vi "Multiprocessing_VI.vi"() -> ()   [LabVIEW 2022 SP3]
uses:
  <vilib>/Analysis/baseanly.llb/Mean (DBL).vi
  <vilib>/DAQmx/read.llb/DAQmx Read (Analog 1D Wfm NChan NSamp).vi
  STOP_GLOBAL.vi
  <vilib>/DAQmx/configure/timing.llb/DAQmx Timing (Sample Clock).vi
  <vilib>/addons/control/pid/pid.llb/PID Gain Schedule (DBL).vi
  <vilib>/DAQmx/miscellaneous.llb/DAQmx Fill In Error Info.vi
  <resource>/objmgr/daqmx.rc
  <vilib>/addons/control/pid/NI_PID_pid.lvlib
  <vilib>/Analysis/NI_AALBase.lvlib
panel:
  out "Angle":dbl
  in  "Voltage 2":dbl
  out "Angle Sensor":dbl[](graph)
  in  "Manual Angle Control":dbl
  out "Voltage":dbl
  out "Voltage Command Output":dbl[](graph)
  out "VoltageSent":dbl
  out "Ball Valve Angle Command":dynamicdata(graph)
  in  "Ignition":bool
  in  "Stepper Voltage":ext format="%_3g"
  out "Chamber Pressure LocalVar":dynamicdata(graph)
  out "PID gains out":T1={"proportional gain (Kc)"=1.0, "integral time (Ti, min)"=0.01, "derivative time (Td, min)"=0.0} {"derivative time (Td, min)" format="%.3f"; "integral time (Ti, min)" format="%.5f"; "proportional gain (Kc)" format="%.3f"}
  out "Process Variable vs Setpoint":dynamicdata(graph)
  out "Output":dbl(slide)=30.8641975308642 scale=0.0..5.067 scale format="%.1f"
  in  "Automatic":bool=TRUE
  out "Servo/Step Voltage":dbl[](array[numeric])
  in  "SP":dbl
  in  "MV":dbl(slide)=30.8641975308642 scale=0.0..5.067 scale format="%.1f"
  in  "Stop All":bool
  out "D.C. Delay":dbl
  out "AI7":dynamicdata(graph)
  out "Time":dbl
  out "Inlet Thermocouple":cluster{dbl[], dbl[]}(graph)
  out "Inlet Thermocouple":dynamicdata(graph)
  out "Flow Meter Thermocouple":dynamicdata(graph)
  out "Flow Meter Thermocouple":cluster{dbl[], dbl[]}(graph)
  out "Supply P. Thermocouple":cluster{dbl[], dbl[]}(graph)
  out "Supply P. Thermocouple":dynamicdata(graph)
  out "Thrust 3":cluster{dbl[], dbl[]}(graph)
  out "Thrust 2":cluster{dbl[], dbl[]}(graph)
  out "Rocket Thrust":cluster{dbl[], dbl[]}(graph)
  out "LC2":dynamicdata(graph)
  out "Rocket Thrust LC1":dynamicdata(graph)
  out "LC3":dynamicdata(graph)
  out "Waiting \nfor Start":bool=TRUE
  in  "Start VI":bool
  out "SampClk.Rate":dbl
  in  "Sample Number":i32=100
  in  "Channel Control":bool[](array[boolean])
  in  "Rate":dbl=1000.0 format="%0.2f"
  out "AI7":cluster{dbl[], dbl[]}(graph)
  out "Vol Flow L/min":dynamicdata(graph)
  out "Process Variable vs Setpoint":cluster{dbl[], dbl[]}[](graph)
  in  "Filename":path=path "C:/1. Rocket Research Project/CollectedData/Plots/TestingData.lvm"
  in  "PID gain schedule":T2(array[cluster])=[{"PID gains"={"proportional gain (Kc)"=1.0, "integral time (Ti, min)"=0.01, "derivative time (Td, min)"=0.0}, "max value"=100.0}] {"max value" format="%.2f"; "PID gains"."derivative time (Td, min)" format="%.3f"; "PID gains"."integral time (Ti, min)" format="%.3f"; "PID gains"."proportional gain (Kc)" format="%.3f"}
  in  "Collect?":bool=TRUE caption="Enable"
  out "Vol Flow":cluster{dbl[], dbl[]}(graph)
  out "Chamber Pressure":cluster{dbl[], dbl[]}(graph)
  out "Inlet Pressure":cluster{dbl[], dbl[]}(graph)
  out "Flow Meter Pressure":cluster{dbl[], dbl[]}(graph)
  out "Supply Pressure":cluster{dbl[], dbl[]}(graph)
  out "Supply Pressure":dynamicdata(graph)
  out "Inlet Pressure":dynamicdata(graph)
  out "Line Pressure":dynamicdata(graph)
  out "Chamber Pressure PSI":dynamicdata(graph)
  out "Output Clock Rate":dbl
  out "For loop iterations":i32
  out "error out":errorcluster
  out "Iterations":i32
  out "Angle Sensor":dynamicdata(graph)
  out "P.T. 5":dynamicdata(graph)
  # "Temperature Channels"
  # "Thrust Channels"
  # "DAQ Configuration"
  # "AI 0 - Supply Pressure"
  # "AI 1 - Flow Meter Pressure"
  # "AI 2 - Inlet Pressure"
  # "AI 3 - Chamber Pressure"
  # "AI 4 - Differential Pressure"
  # "AI 5 - Volumetric Flow"
  # "AI 6 - Angle Sensor"
  # "AI 7"
  # "Load Cell 1 Right"
  # "Load Cell 2 Left"
  # "Thrust Channel 3"
  # "TC1 - Supply P. Thermocouple"
  # "TC2 - Flow Meter Thermocouple"
  # "TC3 - Inlet Thermocouple"
  # "Pressure Channels"
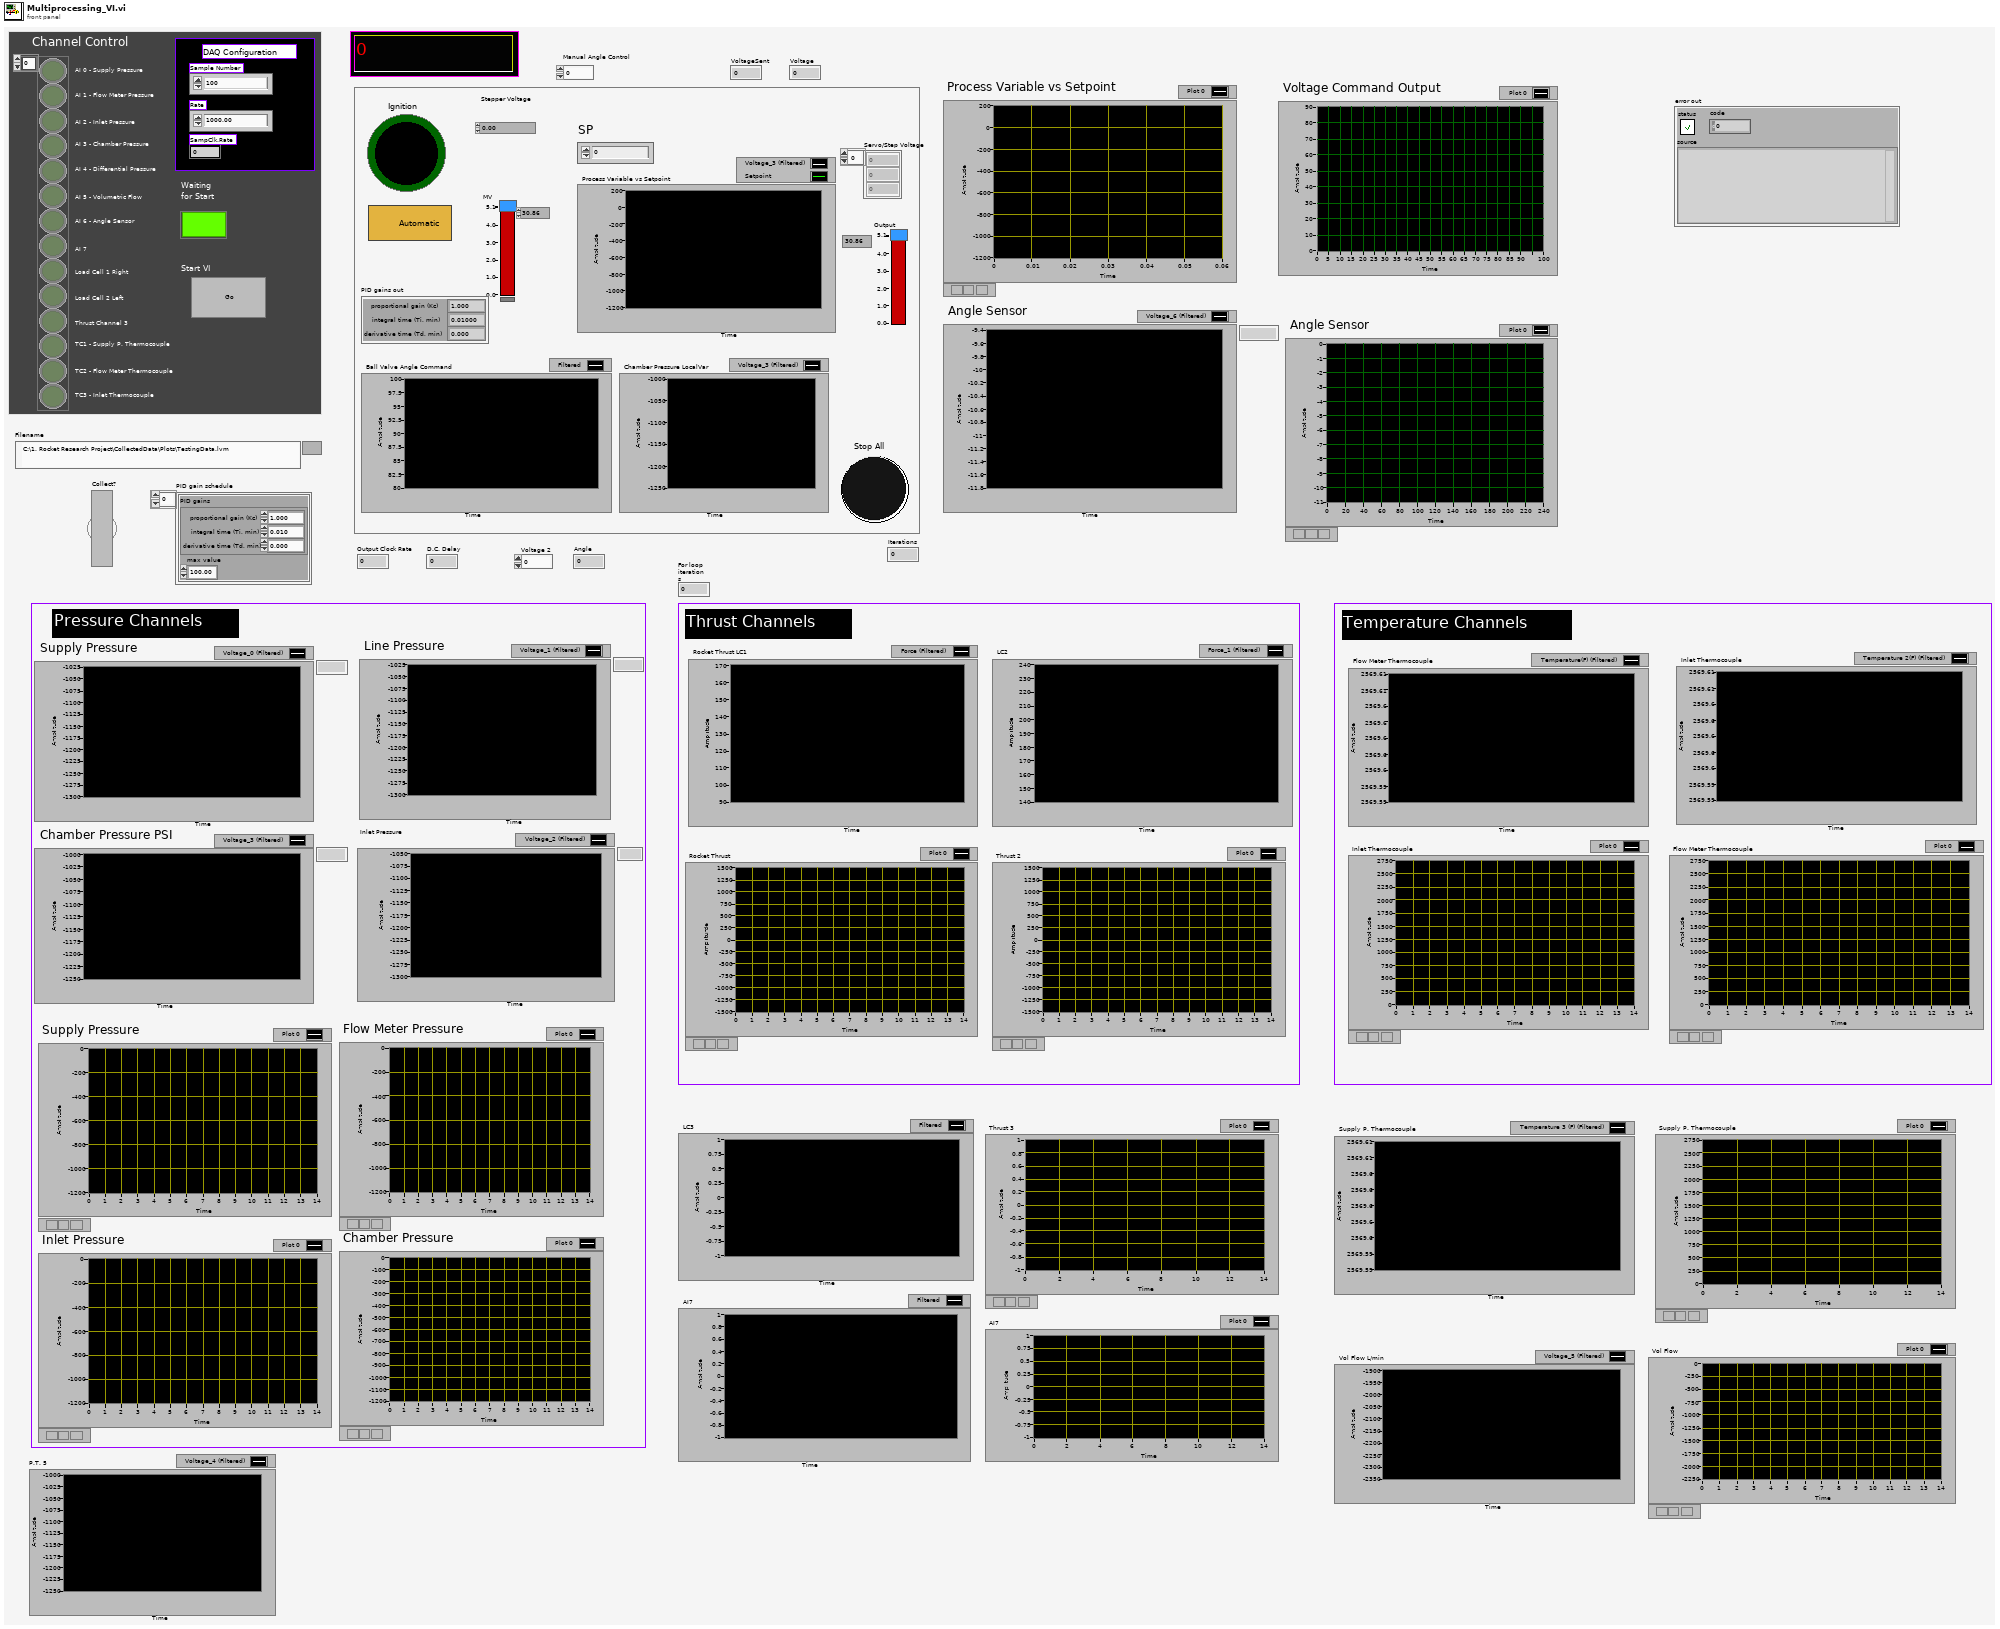
[diagram p1: front panel]
types:
  T1 = cluster{"proportional gain (Kc)":dbl, "integral time (Ti, min)":dbl, "derivative time (Td, min)":dbl}
  T2 = cluster{"PID gains":cluster{"proportional gain (Kc)":dbl, "integral time (Ti, min)":dbl, "derivative time (Td, min)":dbl}, "max value":dbl}[]
  T3 = cluster{"PID gains":cluster{"Kc":dbl, "Ti":dbl, "Td":dbl}, "max value":dbl}[]
  T4 = cluster{"Modulus":dbl, "Number of\nComplete Cycles":dbl}
  T5 = cluster{"Dynamic Data":dynamicdata, "Dynamic Data":dynamicdata, "Dynamic Data":dynamicdata, "Dynamic Data":dynamicdata, "Dynamic Data":dynamicdata, "Dynamic Data":dynamicdata, "Dynamic Data":dynamicdata, "Dynamic Data":dynamicdata, "Dynamic Data":dynamicdata, "Dynamic Data":dynamicdata, "Dynamic Data":dynamicdata, "Dynamic Data":dynamicdata, "Dynamic Data":dynamicdata, "Dynamic Data":dynamicdata}
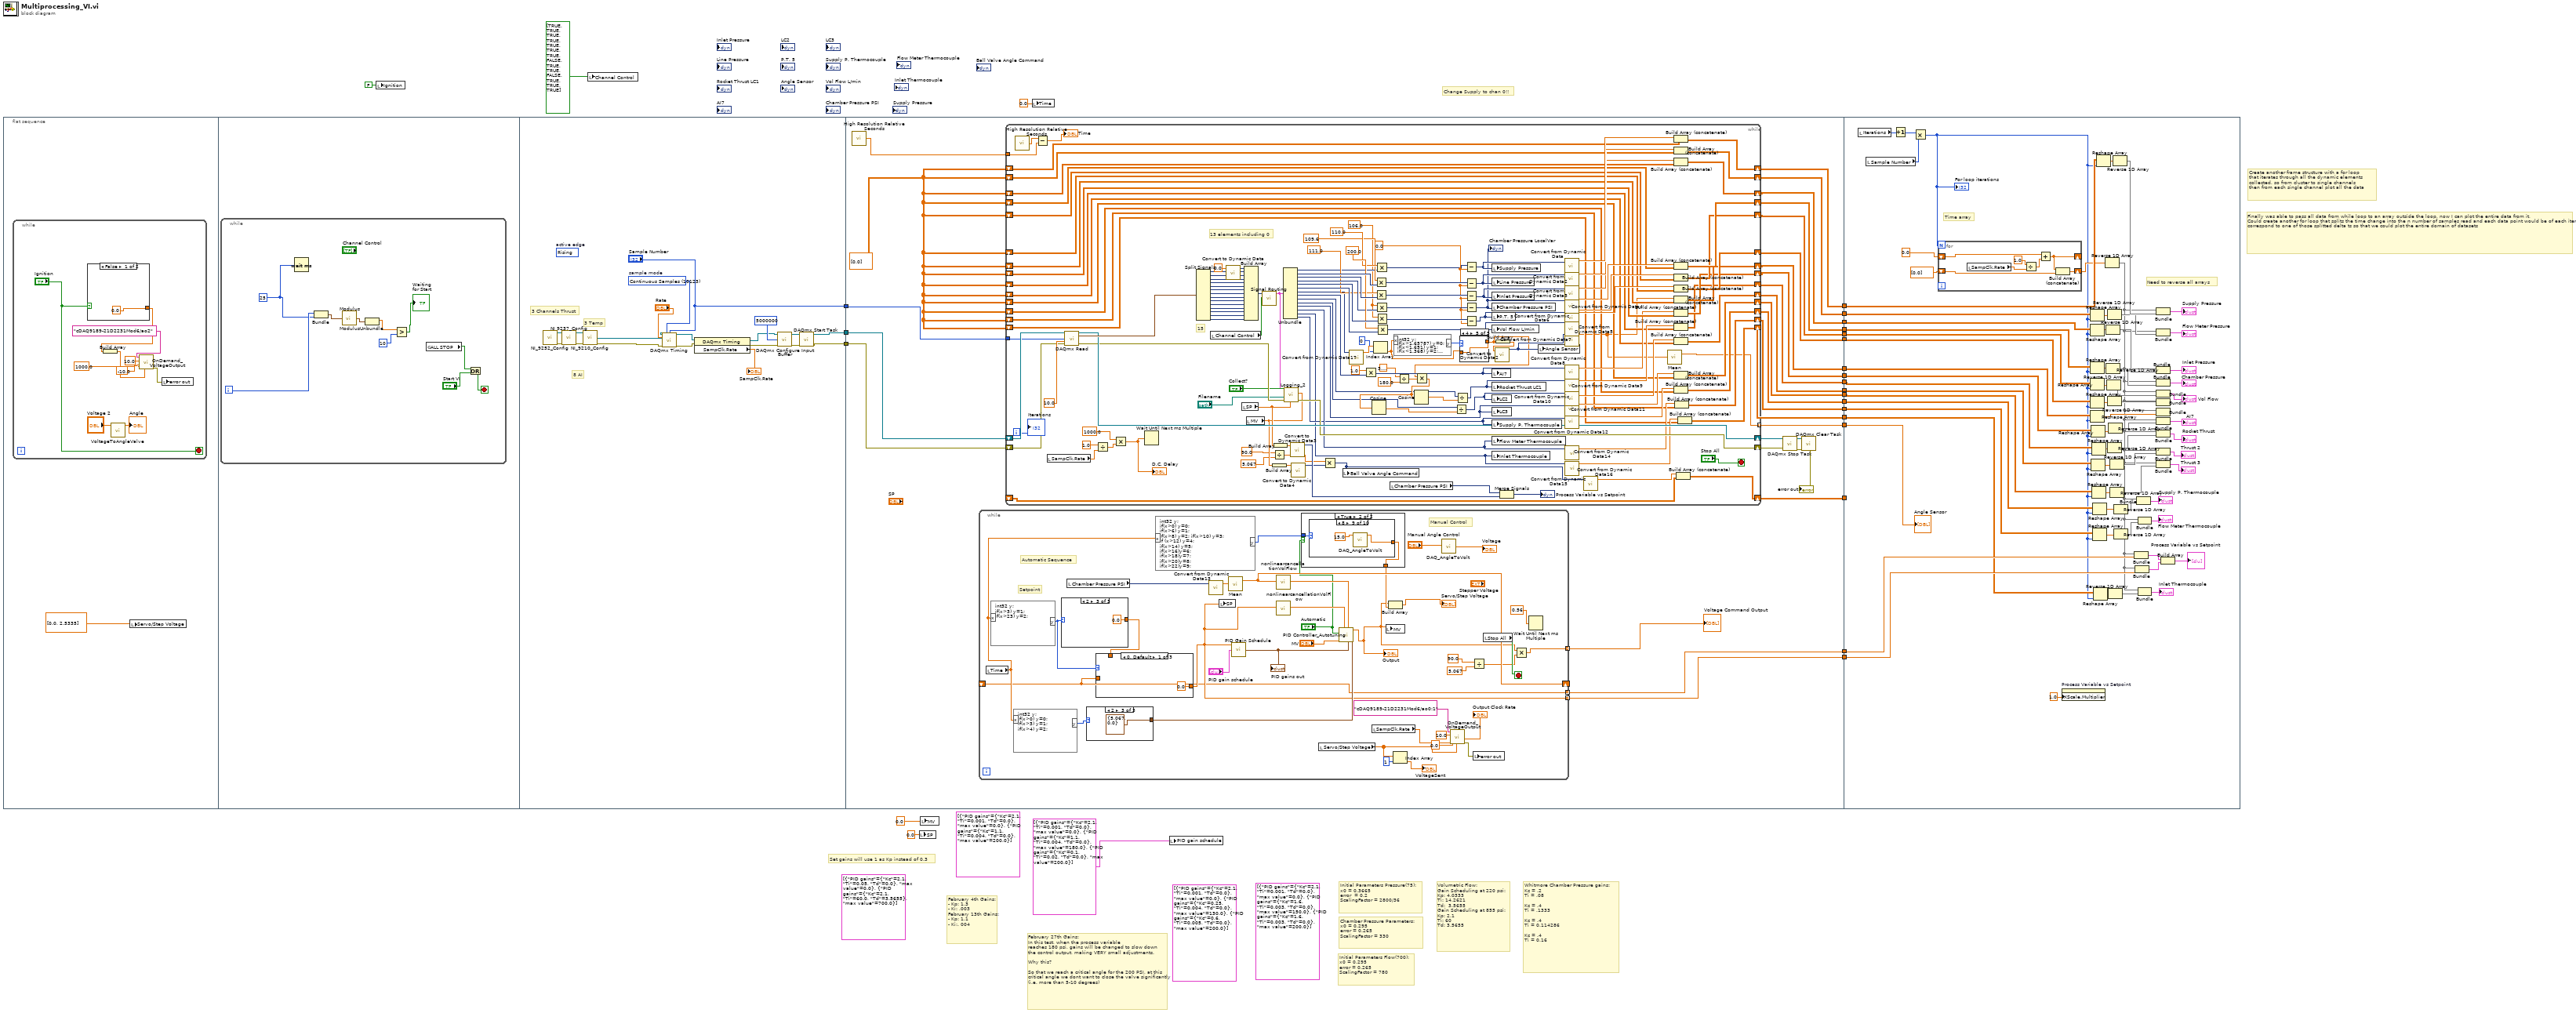
[diagram p0: block diagram]
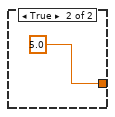
[diagram p2: hidden frame]
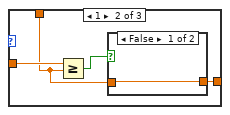
[diagram p3: hidden frame]
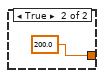
[diagram p4: hidden frame]
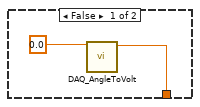
[diagram p6: hidden frame]
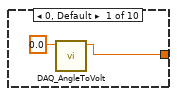
[diagram p7: hidden frame]
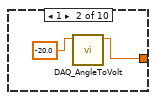
[diagram p8: hidden frame]
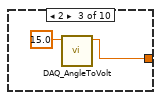
[diagram p9: hidden frame]
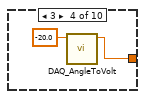
[diagram p10: hidden frame]
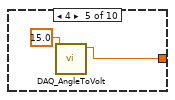
[diagram p11: hidden frame]
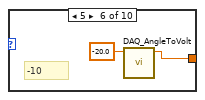
[diagram p12: hidden frame]
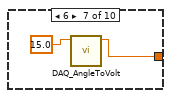
[diagram p13: hidden frame]
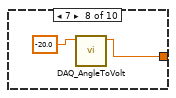
[diagram p14: hidden frame]
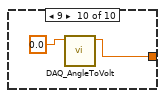
[diagram p15: hidden frame]
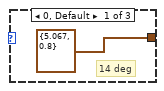
[diagram p16: hidden frame]
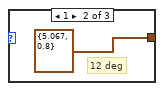
[diagram p17: hidden frame]
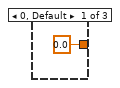
[diagram p18: hidden frame]
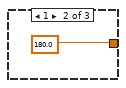
[diagram p19: hidden frame]
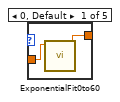
[diagram p20: hidden frame]
diagram:
  (unwired) T3 [{"PID gains"={"Kc"=2.1, "Ti"=0.001, "Td"=0.0}, "max value"=0.0}, {"PID gains"={"Kc"=1.6, "Ti"=0.003, "Td"=0.0}, "max value"=150.0}, {"PID gains"={"Kc"=1.6, "Ti"=0.003, "Td"=0.0}, "max value"=200.0}]
  (unwired) T3 [{"PID gains"={"Kc"=2.1, "Ti"=0.001, "Td"=0.0}, "max value"=0.0}, {"PID gains"={"Kc"=0.25, "Ti"=0.004, "Td"=0.0}, "max value"=130.0}, {"PID gains"={"Kc"=0.6, "Ti"=0.005, "Td"=0.0}, "max value"=200.0}]
  (unwired) T3 [{"PID gains"={"Kc"=2.1, "Ti"=0.05, "Td"=0.0}, "max value"=0.0}, {"PID gains"={"Kc"=2.1, "Ti"=60.0, "Td"=3.5655}, "max value"=700.0}]
  (unwired) T3 [{"PID gains"={"Kc"=2.1, "Ti"=0.001, "Td"=0.0}, "max value"=0.0}, {"PID gains"={"Kc"=1.1, "Ti"=0.004, "Td"=0.0}, "max value"=200.0}]
  # "February 27th Gains:\nIn this test, when the process variable\nreaches 180 psi, gains will be changed to slow down\nthe control output, making VERY small adjustments.\n\nWhy this? \n\nSo that we reach a critical angle for the 200 PSI, at this\ncritical angle we dont want to close the valve significantly\n(i.e. more than 5-10 degrees)"
  # "February 4th Gains:\n- Kp: 1.3\n- Ki: .003\nFebruary 13th Gains:\n- Kp: 1.1\n- Ki:. 004"
  # "Set gains will use 1 as Kp instead of 0.3"
  # "Whitmore Chamber Pressure gains:\nKc = .2\nTi = .08\n\nKc = .4\nTi = .1333\n\nKc = .4\nTi = 0.114286\n\nKc = .4\nTi = 0.16"
  # "Chamber Pressure Parameters:\nx0 = 0.295\nerror = 0.265\nScalingFactor = 330"
  # "Volumetric Flow:\nGain Scheduling at 220 psi:\nKp: 4.0333\nTi: 14.2621\nTd:  3.5655\nGain Scheduling at 855 psi:\nKp: 2.1\nTi: 60\nTd: 3.5655"
  # "Initial Parameters Flow(700):\nx0 = 0.295\nerror = 0.265\nScalingFactor = 780"
  # "Initial Parameters Pressure(75):\nx0 = 0.3665\nerror  = 0.2\nScalingFactor = 2800/36"
  # "Change Supply to chan 0!!"
  # "Finally was able to pass all data from while loop to an array outside the loop, now I can plot the entire data from it, \nCould create another for loop that splits the time change into the n number of samples read and each data point would be of each iteration would correspond to one of those splitted delta ts so that we could plot the entire domain of datasets"
  # "Create another frame structure with a for loop\nthat iterates through all the dynamic elements\ncollected, so from cluster to single channels\nthen from each single channel plot all the data"
  n1 = flat-sequence {
    tunnel: [w62] -> w26
    tunnel: [w51] -> w25
    tunnel: ["Sample Number"] -> w5
    tunnel: w26 -> [w98]
    tunnel: w25 -> [w97]
    tunnel: [w90] -> w24
    tunnel: [w89] -> w22
    tunnel: [w88] -> w21
    tunnel: [w87] -> w20
    tunnel: [w86] -> w19
    tunnel: [w85] -> w18
    tunnel: [w84] -> w17
    tunnel: [w83] -> w16
    tunnel: [w82] -> w15
    tunnel: [w81] -> w14
    tunnel: [w80] -> w13
    tunnel: [w79] -> w12
    tunnel: [w78] -> w10
    tunnel: [w77] -> w9
    tunnel: [w75] -> w7
    tunnel: [w74] -> w6
    tunnel: w5 -> [w73]
    tunnel: [w72] -> w3
    tunnel: [w70] -> w2
    tunnel: w24 -> [w390]
    tunnel: w22 -> [w389]
    tunnel: w21 -> [w388]
    tunnel: w20 -> [w387]
    tunnel: w19 -> [w386]
    tunnel: w18 -> [w385]
    tunnel: w17 -> [w384]
    tunnel: w16 -> [w382]
    tunnel: w15 -> [w381]
    tunnel: w14 -> [w380]
    tunnel: w13 -> [w379]
    tunnel: w12 -> [w378]
    tunnel: w10 -> [w373]
    tunnel: w9 -> [w372]
    tunnel: w7 -> [w347]
    tunnel: w6 -> [w346]
    tunnel: w3 -> [_]
    tunnel: w2 -> [w328]
    frame #0 {
      n2 = while {
        stop <- "Ignition" stop-if-true
        n3 = case shown="False" "Ignition" {
          tunnel: [0.0 ("element") 5.0 ("element")] -> w37
          frame False {
          }
          frame True {
          }
        }
        n4 = Build Array(w37) -> (w38:dbl[])
        n5 = call "VoltageToAngleValve.vi"("Voltage"="Voltage 2") -> ("Angle"=→"Angle":dbl)  [unwired: 10 in]
        n6 = call "OnDemand_VoltageOutput.vi"("Channel Array"=w38, "SampClk.Rate 2"=1000.0, "minimum voltage"=-10.0, "maximum voltage"=10.0, "physical channels"="cDAQ9189-21D2231Mod6/ao2") -> ("error out"=w36:errorcluster)  [unwired: 4 in, 2 out]
        n7 = local write "error out"(w36) -> ()
      }
      n8 = local write "Servo/Step Voltage"(dbl[] [0.0, 2.5335] ("Servo/Step Voltage")) -> ()
    }
    frame #1 {
      n9 = while {
        i -> [w50]
        stop <- w42 stop-if-true
        w41 = u32 25 ("milliseconds to wait")
        n10 = Wait (ms)(milliseconds to wait=w41) -> ()  [unwired: 1 out]
        n11 = Bundle(w50, "milliseconds to wait"=w41) -> (w49:cluster{i32, "milliseconds to wait":u32})  [unwired: 1 in]
        n12 = call "Modulus.vi"("Input"=w49) -> ("Output"=w48:T4)
        n13 = call "Modulus.vi"() -> ()  [unwired: 1 in, 1 out]
        n14 = Unbundle(w48) -> ("Modulus"=w47:dbl)  [unwired: 1 out]
        n15 = Greater?(x=w47, y=u32 10 ("milliseconds to wait")) -> (0:→"Waiting \nfor Start":bool)
        n16 = global read "STOP_GLOBAL.vi" "ALL STOP"() -> (w44:bool)
        n17 = Or(x=w44, y="Start VI") -> (x .or. y?=w42:bool)
      }
    }
    frame #2 {
      w53 = 10123 items=["Finite Samples"=10178, "Continuous Samples"=10123, "Hardware Timed Single Point"=12522]  # sample mode
      (unwired) 10280 items=["Rising"=10280, "Falling"=10171]  # active edge
      # "3 Temp"
      # "8 AI"
      # "3 Channels Thrust"
      n18 = call "NI_9252_Config.vi"() -> ("error out"=w60:errorcluster, "task out"=w61:refnum<k21>)  [unwired: 10 in]
      n19 = call "NI 9237_Config.vi"("error in"=w60, "task in"=w61) -> ("error out"=w69:errorcluster, "task out"=w68:refnum<k21>)  [unwired: 8 in]
      n20 = call "NI_9210_Config.vi"("error in"=w69, "task in"=w68) -> ("error out"=w56:errorcluster, "task out"=w58:refnum<k21>)  [unwired: 8 in]
      n21 = call-poly <vilib>:"DAQmx Timing.vi"("task/channels in"=w58, "sample mode"=w53, "samples per channel"="Sample Number", "rate"="Rate", "error in"=w56) -> ("task out"=w54:refnum<k21>, "error out"=w55:errorcluster)  [unwired: 9 in]
      n22 = property class="DAQmx Timing"(reference=w54, error in=w55) -> (reference out=w52:refnum<k21>, error out=w65:errorcluster, "SampClk.Rate"=→"SampClk.Rate":dbl)
      n23 = call <vilib>:"DAQmx Configure Input Buffer.vi"("task/channels in"=w52, "buffer size (in samples per channel)"=u32 5000000, "error in"=w65) -> ("task out"=w67:refnum<k21>, "error out"=w66:errorcluster)  [unwired: 11 in]
      n24 = call <vilib>:"DAQmx Start Task.vi"("task/channels in"=w67, "error in"=w66) -> ("task out"=w62:refnum<k21>, "error out"=w51:errorcluster)  [unwired: 12 in]
    }
    frame #3 {
      w76 = dbl[][] [[0.0]]
      n25 = call <vilib>:"High Resolution Relative Seconds.vi"() -> ("relative seconds"=w96:dbl)
      n26 = while {
        shift-right: [w128] -> _
        shift-left: _ -> [w99]
        tunnel: [w99] -> w78 mode=indexing
        tunnel: [w100] -> w77 mode=indexing
        tunnel: [w107] -> w71 mode=indexing
        stop <- w131 stop-if-true
        # "Manual Control"
        # "Automatic Sequence"
        # "Setpoint"
        n27 = local read "Time"() -> (w116:dbl)
        n28 = formula code="int32 y;\nif(x>3) y=1;\nif(x>23) y=2;"("x"=w116) -> ("y"=w102:i32)
        n29 = formula code="int32 y;\nif(x>0) y=0;\nif(x>3) y=1;\nif(x>4) y=2;"("x"=w116) -> ("y"=w127:i32)
        n30 = case shown="2" w102 {
          tunnel: [0.0 ("SP") 180.0 ("SP") 0.0 ("SP")] -> w101
          frame 0, Default {
          }
          frame 1 {
          }
          frame 2 {
          }
        }
        n31 = local read "Chamber Pressure PSI"() -> (w118:dynamicdata)
        n32 = case shown="2" w127 {
          tunnel: [cluster{"output high":dbl, "output low":dbl} {"output high"=5.067, "output low"=0.8} ("output range") cluster{"output high":dbl, "output low":dbl} {"output high"=5.067, "output low"=0.8} ("output range") cluster{"output high":dbl, "output low":dbl} {"output high"=5.067, "output low"=0.0} ("output range")] -> w126
          frame 0, Default {
            # "14 deg"
          }
          frame 1 {
            # "12 deg"
          }
          frame 2 {
          }
        }
        n33 = case shown="0, Default" w102 {
          tunnel: w99 -> [_ w140 _]
          tunnel: w101 -> [_ w138 w143]
          tunnel: [0.0 ("SP") w137 w143] -> w100
          frame 0, Default {
          }
          frame 1 {
            n34 = Greater Or Equal?(x=w140, y=w138) -> (x >= y?=w139:bool)
            n35 = case shown="False" w139 {
              tunnel: w138 -> [w141 _]
              tunnel: [w141 200.0 ("SP")] -> w137
              frame False {
              }
              frame True {
              }
            }
          }
          frame 2 {
          }
        }
        n36 = formula code="int32 y;\nif(x>0) y=0;\nif(x>6) y=1;\nif(x>8) y=2; if(x>10) y=3;\nif (x>12) y=4;\nif(x>14) y=5;\nif(x>16)y=6;\nif(x>18)y=7;\nif(x>20)y=8;\nif(x>22)y=9;"("x"=w116) -> ("y"=w103:i32)
        n37 = call "Convert from Dynamic Data13"("Dynamic Data Type"=w118) -> ("Array"=w129:dbl[])  [unwired: 3 in]
        n38 = local write "SP"(w100) -> ()
        n39 = call-poly <vilib>:"Mean.vi"("X"=w129) -> ("mean"=w128:dbl)  [unwired: 1 out]
        n40 = call-poly <vilib>:"PID Gain Schedule.vi"("PID gain schedule"="PID gain schedule", "gain scheduling value"=w100) -> ("PID gains out"=w134:T1)  [unwired: 2 in, 1 out]
        "PID gains out" <- w134
        n41 = call "nonlinearcancellationVolFlow.vi"("input variable"=w128) -> ("MVT Process Variable"=w130:dbl)  [unwired: 10 in]
        n42 = call "nonlinearcancellationVolFlow.vi"("input variable"=w100) -> ("MVT Process Variable"=w132:dbl)  [unwired: 10 in]
        n43 = case shown="True" "Automatic" {
          tunnel: [w144 w147] -> w110
          tunnel: w103 -> [_ w146]
          frame False {
            n44 = call "DAQ_AngleToVolt.vi"("Angle"=0.0 ("Voltage")) -> ("Voltage"=w144:dbl)  [unwired: 10 in]
          }
          frame True {
            n45 = case shown="8" w146 {
              tunnel: [w149 w150 w152 w155 w156 w159 w160 w162 w164 w166] -> w147
              frame 0, Default {
                n46 = call "DAQ_AngleToVolt.vi"("Angle"=0.0) -> ("Voltage"=w149:dbl)  [unwired: 10 in]
              }
              frame 1 {
                n47 = call "DAQ_AngleToVolt.vi"("Angle"=-20.0 ("x")) -> ("Voltage"=w150:dbl)  [unwired: 10 in]
              }
              frame 2 {
                n48 = call "DAQ_AngleToVolt.vi"("Angle"=15.0) -> ("Voltage"=w152:dbl)  [unwired: 10 in]
              }
              frame 3 {
                n49 = call "DAQ_AngleToVolt.vi"("Angle"=-20.0) -> ("Voltage"=w155:dbl)  [unwired: 10 in]
              }
              frame 4 {
                n50 = call "DAQ_AngleToVolt.vi"("Angle"=15.0) -> ("Voltage"=w156:dbl)  [unwired: 10 in]
              }
              frame 5 {
                # "-10"
                n51 = call "DAQ_AngleToVolt.vi"("Angle"=-20.0) -> ("Voltage"=w159:dbl)  [unwired: 10 in]
              }
              frame 6 {
                n52 = call "DAQ_AngleToVolt.vi"("Angle"=15.0) -> ("Voltage"=w160:dbl)  [unwired: 10 in]
              }
              frame 7 {
                n53 = call "DAQ_AngleToVolt.vi"("Angle"=-20.0) -> ("Voltage"=w162:dbl)  [unwired: 10 in]
              }
              frame 8 {
                n54 = call "DAQ_AngleToVolt.vi"("Angle"=15.0) -> ("Voltage"=w164:dbl)  [unwired: 10 in]
              }
              frame 9 {
                n55 = call "DAQ_AngleToVolt.vi"("Angle"=0.0) -> ("Voltage"=w166:dbl)  [unwired: 10 in]
              }
            }
          }
        }
        n56 = local read "Servo/Step Voltage"() -> (w115:dbl[])
        n57 = call "PID Controller_Autotuning.vi"("output range"=w126, "PID gains in"=w134, "process variable"=w130, "setpoint"=w132, "manipulated variable"="MV", "Automatic"="Automatic") -> ("output"=w105:dbl)  [unwired: 4 in, 1 out]
        "Output" <- w105
        n58 = local read "SampClk.Rate"() -> (w124:dbl)
        n59 = local write "MV"(w105) -> ()
        n60 = Build Array(w105, w110) -> (→"Servo/Step Voltage":dbl[])
        n61 = Index Array(array=w115, index=1) -> (element=→"VoltageSent":dbl)
        n62 = call "DAQ_AngleToVolt.vi"("Angle"="Manual Angle Control") -> ("Voltage"=→"Voltage":dbl)  [unwired: 10 in]
        n63 = call "OnDemand_VoltageOutput.vi"("Channel Array"=w115, "SampClk.Rate 2"=w124, "minimum voltage"=0.0, "maximum voltage"=10.0, "physical channels"="cDAQ9189-21D2231Mod6/ao0:1") -> ("error out"=w123:errorcluster, "SampClk.Rate"=→"Output Clock Rate":dbl)  [unwired: 4 in, 1 out]
        n64 = Divide(x=90.0, y=5.067) -> (x/y=w106:dbl)
        n65 = local write "error out"(w123) -> ()
        n66 = local read "Stop All"() -> (w131:bool)
        n67 = Multiply(x=w105, y=w106) -> (x*y=w107:dbl)
        n68 = Wait Until Next ms Multiple(millisecond multiple=0.56 ("x")) -> ()  [unwired: 1 out]
      }
      "Voltage Command Output" <- w71
      n69 = while {
        shift-right: [w314] -> w92
        shift-left: w98 -> [w316]
        shift-right: [w292] -> w91
        shift-left: w97 -> [w315]
        shift-right: [w205] -> w90
        shift-left: w76 -> [w254]
        tunnel: w96 -> [w289]
        shift-right: [w284] -> w89
        shift-left: w76 -> [w174]
        shift-right: [w280] -> w88
        shift-left: w76 -> [w281]
        shift-right: [w278] -> w87
        shift-left: w76 -> [w279]
        shift-right: [w276] -> w86
        shift-left: w76 -> [w275]
        shift-right: [w273] -> w85
        shift-left: w76 -> [w271]
        shift-right: [w272] -> w84
        shift-left: w76 -> [w270]
        shift-right: [w269] -> w83
        shift-left: w76 -> [w268]
        shift-right: [w264] -> w82
        shift-left: w76 -> [w263]
        shift-right: [w262] -> w81
        shift-left: w76 -> [w261]
        shift-right: [w259] -> w80
        shift-left: w76 -> [w258]
        shift-right: [w256] -> w79
        shift-left: w76 -> [w255]
        shift-right: [w233] -> w75
        shift-left: w76 -> [w232]
        shift-right: [w229] -> w74
        shift-left: w76 -> [w230]
        tunnel: w73 -> [w226]
        shift-right: [w200] -> w72
        shift-left: _ -> [w201]
        tunnel: [w175] -> w70 mode=indexing
        i -> [w291]
        stop <- "Stop All" stop-if-true
        w196 = 106.0 ("x")
        w218 = 0.0 ("y")
        # "13 elements including 0"
        # "15"
        n70 = call <vilib>:"High Resolution Relative Seconds.vi"() -> ("relative seconds"=w290:dbl)
        n71 = Subtract(x=w290, y=w289) -> (x-y=→"Time":dbl)
        n72 = local read "SampClk.Rate"() -> (w251:dbl)
        n73 = call-poly <vilib>:"DAQmx Read.vi"("task/channels in"=w316, "number of samples per channel"=w226, "timeout"=10.0, "error in"=w315) -> ("task out"=w314:refnum<k21>, "data"=w317:waveform(dbl)[], "error out"=w294:errorcluster)  [unwired: 9 in]
        n74 = Divide(x=1.0, y=w251) -> (x/y=w250:dbl)
        n75 = Multiply(x=1000.0, y=w250) -> (x*y=w248:dbl)
        "D.C. Delay" <- w248
        n76 = Wait Until Next ms Multiple(millisecond multiple=w248) -> ()  [unwired: 1 out]
        n77 = Split Signals(w317) -> (w308:dynamicdata, w313:dynamicdata, w312:dynamicdata, w311:dynamicdata, w310:dynamicdata, w309:dynamicdata, w307:dynamicdata, w306:dynamicdata, w305:dynamicdata, w304:dynamicdata, w303:dynamicdata, w300:dynamicdata, w236:dynamicdata, w235:dynamicdata)  [unwired: 14 in]
        n78 = local read "Channel Control"() -> (w299:bool[])
        n79 = call "Convert to Dynamic Data"("Double"=0.0) -> ("Dynamic Data Type"=w301:dynamicdata)  [unwired: 3 in]
        n80 = local read "SP"() -> (w216:dbl)
        n81 = Build Array(w301, w308, w313, w312, w311, w310, w309, w307, w306, w305, w304, w303, w300, w236, w235) -> (w298:dynamicdata[])
        n82 = local read "MV"() -> (w211:dbl)
        n83 = call "Signal Routing.vi"("Boolean Array"=w299, "Data In"=w298) -> ("Output"=w225:T5)  [unwired: 9 in]
        n84 = Build Array(w211) -> (w210:dbl[])
        n85 = Divide(x=90.0, y=5.067) -> (x/y=w199:dbl)
        n86 = Build Array(w216) -> (w215:dbl[])
        n87 = Unbundle(w225) -> ("Dynamic Data"=w204:dynamicdata, "Dynamic Data"=w297:dynamicdata, "Dynamic Data"=w296:dynamicdata, "Dynamic Data"=w217:dynamicdata, "Dynamic Data"=w295:dynamicdata, "Dynamic Data"=w228:dynamicdata, "Dynamic Data"=w189:dynamicdata, "Dynamic Data"=w247:dynamicdata, "Dynamic Data"=w181:dynamicdata, "Dynamic Data"=w180:dynamicdata, "Dynamic Data"=w178:dynamicdata, "Dynamic Data"=w224:dynamicdata, "Dynamic Data"=w222:dynamicdata, "Dynamic Data"=w223:dynamicdata)
        n88 = call "Logging_2.vi"("Voltage Command"=w211, "Setpoint"=w216, "error in"=w294, "Filename"="Filename", "Enable"="Collect?", "output cluster"=w225) -> ("error out"=w292:errorcluster)  [unwired: 5 in]
        n89 = call "Convert to Dynamic Data3"("Array"=w215) -> ("Dynamic Data Type"=w214:dynamicdata)  [unwired: 3 in]
        n90 = call "Convert to Dynamic Data4"("Array"=w210) -> ("Dynamic Data Type"=w209:dynamicdata)  [unwired: 3 in]
        n91 = Multiply(x=w199, y=w209) -> (x*y=w203:dynamicdata)
        n92 = local write "Ball Valve Angle Command"(w203) -> ()
        n93 = call "Convert from Dynamic Data17"("Dynamic Data Type"=w189) -> ("Array"=w194:dbl[])  [unwired: 3 in]
        n94 = Multiply(x=1.0, y=w247) -> (x*y=w245:dynamicdata)
        n95 = Index Array(array=w194, index=0) -> (element=w177:dbl)
        n96 = Multiply(x=109.6, y=w297) -> (x*y=w243:dynamicdata)
        n97 = Multiply(x=111.0, y=w296) -> (x*y=w244:dynamicdata)
        n98 = Multiply(x=110.0, y=w204) -> (x*y=w242:dynamicdata)
        n99 = Multiply(x=w196, y=w217) -> (x*y=w238:dynamicdata)
        n100 = Multiply(x=w196, y=w295) -> (x*y=w220:dynamicdata)
        n101 = Multiply(x=200.0, y=w228) -> (x*y=w221:dynamicdata)
        n102 = local read "Chamber Pressure PSI"() -> (w212:dynamicdata)
        n103 = formula code="int32 y;\nif(x>1.65787) y=0;\nif(x<1.651) y=1;\nif(x<1.368) y=2;\nif(x>1.935) y=3;\nif(x<1.36) y=4;"("x"=w177) -> ("y"=w195:i32)
        n104 = Divide(x=3.141592653589793, y=180.0 ("x")) -> (x/y=w185:dbl)
        n105 = case shown="4" w195 {
          tunnel: w177 -> [w320 w322 w324 w326 w327]
          tunnel: [w319 w321 w323 w325 w327] -> w184
          frame 0, Default {
            n106 = call "ExponentialFit0to60.vi"("voltage"=w320) -> ("angle"=w319:dbl)  [unwired: 10 in]
          }
          frame 1 {
            n107 = call "PolyFit0to-60.vi"("input variable"=w322) -> ("output variable"=w321:dbl)  [unwired: 10 in]
          }
          frame 2 {
            n108 = call "PolyFit-60to-90.vi"("Voltage"=w324) -> ("Angle"=w323:dbl)  [unwired: 10 in]
          }
          frame 3 {
            n109 = call "PolynomialFit60to90.vi"("voltage"=w326) -> ("Angle"=w325:dbl)  [unwired: 10 in]
          }
          frame 4 {
          }
        }
        n110 = Multiply(x=w184, y=w185) -> (x*y=w183:dbl)
        n111 = Cosine(x=w183) -> (cos(x)=w190:dbl)
        n112 = Cosine(x=w183) -> (cos(x)=w191:dbl)
        n113 = Divide(x=w180, y=w190) -> (x/y=w179:dynamicdata)
        n114 = Divide(x=w181, y=w191) -> (x/y=w182:dynamicdata)
        n115 = Subtract(x=w242, y=w218) -> (x-y=w241:dynamicdata)
        n116 = Subtract(x=w243, y=w218) -> (x-y=w240:dynamicdata)
        n117 = Subtract(x=w244, y=w218) -> (x-y=w239:dynamicdata)
        n118 = Subtract(x=w238, y=w218) -> (x-y=w237:dynamicdata)
        "Chamber Pressure LocalVar" <- w237
        n119 = Subtract(x=w220, y=w218) -> (x-y=w219:dynamicdata)
        n120 = local write "Supply Pressure"(w241) -> ()
        n121 = local write "Line Pressure"(w240) -> ()
        n122 = local write "Inlet Pressure"(w239) -> ()
        n123 = local write "Chamber Pressure PSI"(w237) -> ()
        n124 = local write "P.T. 5"(w219) -> ()
        n125 = local write "Vol Flow L/min"(w221) -> ()
        n126 = local write "AI7"(w245) -> ()
        n127 = local write "Rocket Thrust LC1"(w182) -> ()
        n128 = local write "LC2"(w179) -> ()
        n129 = local write "LC3"(w178) -> ()
        n130 = local write "Supply P. Thermocouple"(w223) -> ()
        n131 = local write "Flow Meter Thermocouple"(w224) -> ()
        n132 = local write "Inlet Thermocouple"(w222) -> ()
        n133 = Build Array(w184) -> (w192:dbl[])
        n134 = call "Convert to Dynamic Data2"("Array"=w192) -> ("Dynamic Data Type"=w188:dynamicdata)  [unwired: 3 in]
        n135 = Merge Signals(w212, w214) -> (→"Process Variable vs Setpoint":dynamicdata)
        n136 = local write "Angle Sensor"(w188) -> ()
        n137 = call "Convert from Dynamic Data"("Dynamic Data Type"=w241) -> ("Array"=w288:dbl[])  [unwired: 3 in]
        n138 = call "Convert from Dynamic Data2"("Dynamic Data Type"=w240) -> ("Array"=w285:dbl[])  [unwired: 3 in]
        n139 = call "Convert from Dynamic Data3"("Dynamic Data Type"=w239) -> ("Array"=w283:dbl[])  [unwired: 3 in]
        n140 = call "Convert from Dynamic Data4"("Dynamic Data Type"=w237) -> ("Array"=w282:dbl[])  [unwired: 3 in]
        n141 = call "Convert from Dynamic Data6"("Dynamic Data Type"=w219) -> ("Array"=w274:dbl[])  [unwired: 3 in]
        n142 = call "Convert from Dynamic Data5"("Dynamic Data Type"=w221) -> ("Array"=w277:dbl[])  [unwired: 3 in]
        n143 = call "Convert from Dynamic Data7"("Dynamic Data Type"=w188) -> ("Array"=w176:dbl[])  [unwired: 3 in]
        n144 = call "Convert from Dynamic Data8"("Dynamic Data Type"=w245) -> ("Array"=w267:dbl[])  [unwired: 3 in]
        n145 = call "Convert from Dynamic Data9"("Dynamic Data Type"=w182) -> ("Array"=w266:dbl[])  [unwired: 3 in]
        n146 = call "Convert from Dynamic Data10"("Dynamic Data Type"=w179) -> ("Array"=w265:dbl[])  [unwired: 3 in]
        n147 = call "Convert from Dynamic Data11"("Dynamic Data Type"=w178) -> ("Array"=w260:dbl[])  [unwired: 3 in]
        n148 = call "Convert from Dynamic Data12"("Dynamic Data Type"=w223) -> ("Array"=w257:dbl[])  [unwired: 3 in]
        n149 = call "Convert from Dynamic Data14"("Dynamic Data Type"=w224) -> ("Array"=w234:dbl[])  [unwired: 3 in]
        n150 = call "Convert from Dynamic Data15"("Dynamic Data Type"=w222) -> ("Array"=w231:dbl[])  [unwired: 3 in]
        n151 = call "Convert from Dynamic Data16"("Dynamic Data Type"=w203) -> ("Array"=w202:dbl[])  [unwired: 3 in]
        n152 = call-poly <vilib>:"Mean.vi"("X"=w176) -> ("mean"=w175:dbl)  [unwired: 1 out]
        n153 = Build Array (concatenate)(w288, w254) -> (w205:dbl[][])
        n154 = Build Array (concatenate)(w285, w174) -> (w284:dbl[][])
        n155 = Build Array (concatenate)(w283, w281) -> (w280:dbl[][])
        n156 = Build Array (concatenate)(w282, w279) -> (w278:dbl[][])
        n157 = Build Array (concatenate)(w277, w275) -> (w276:dbl[][])
        n158 = Build Array (concatenate)(w274, w271) -> (w273:dbl[][])
        n159 = Build Array (concatenate)(w176, w270) -> (w272:dbl[][])
        n160 = Build Array (concatenate)(w267, w268) -> (w269:dbl[][])
        n161 = Build Array (concatenate)(w266, w263) -> (w264:dbl[][])
        n162 = Build Array (concatenate)(w265, w261) -> (w262:dbl[][])
        n163 = Build Array (concatenate)(w260, w258) -> (w259:dbl[][])
        n164 = Build Array (concatenate)(w257, w255) -> (w256:dbl[][])
        n165 = Build Array (concatenate)(w234, w232) -> (w233:dbl[][])
        n166 = Build Array (concatenate)(w202, w201) -> (w200:dbl[][])
        n167 = Build Array (concatenate)(w231, w230) -> (w229:dbl[][])
        "Iterations" <- w291
      }
      n168 = call <vilib>:"DAQmx Stop Task.vi"("task/channels in"=w92, "error in"=w91) -> ("task out"=w95:refnum<k21>, "error out"=w94:errorcluster)  [unwired: 12 in]
      n169 = call <vilib>:"DAQmx Clear Task.vi"("task in"=w95, "error in"=w94) -> ("error out"=→"error out":errorcluster)  [unwired: 13 in]
    }
    frame #4 {
      # "Time array"
      # "Need to reverse all arrays"
      n170 = local read "Iterations"() -> (w395:i32)
      n171 = local read "Sample Number"() -> (w331:i32)
      n172 = Increment(x=w395) -> (x+1=w394:i32)
      n173 = Multiply(x=w394, y=w331) -> (x*y=w330:i32)
      "For loop iterations" <- w330
      n174 = for {
        N: w330 -> [_]
        shift-right: [w398] -> _
        shift-left: 0.0 -> [w399]
        shift-right: [w397] -> w368
        shift-left: dbl[] [0.0] -> [w396]
        n175 = local read "SampClk.Rate"() -> (w401:dbl)
        n176 = Divide(x=1.0, y=w401) -> (x/y=w400:dbl)
        n177 = Add(x=w399, y=w400) -> (x+y=w398:dbl)
        n178 = Build Array (concatenate)(w398, w396) -> (w397:dbl[])
      }
      n179 = property on="Process Variable vs Setpoint" class="XYGraph (strict)"("XScale.Multiplier"=1.0 ("X Scale.Offset and Multiplier:Multiplier")) -> ()  [unwired: 2 in, 2 out]
      n180 = Reshape Array(w389, w330) -> (w364:dbl[])
      n181 = Reshape Array(w388, w330) -> (w362:dbl[])
      n182 = Reshape Array(w387, w330) -> (w360:dbl[])
      n183 = Reshape Array(w386, w330) -> (w358:dbl[])
      n184 = Reshape Array(w385, w330) -> (w356:dbl[])
      n185 = Reshape Array(w384, w330) -> (w383:dbl[])
      n186 = Reshape Array(w382, w330) -> (w353:dbl[])
      n187 = Reshape Array(w380, w330) -> (w337:dbl[])
      n188 = Reshape Array(w381, w330) -> (w345:dbl[])
      n189 = Reshape Array(w379, w330) -> (w334:dbl[])
      n190 = Reshape Array(w378, w330) -> (w350:dbl[])
      n191 = Reshape Array(w347, w330) -> (w343:dbl[])
      n192 = Reshape Array(w346, w330) -> (w338:dbl[])
      n193 = Reshape Array(w390, w330) -> (w366:dbl[])
      n194 = Reverse 1D Array(array=w368) -> (reversed array=w329:dbl[])
      n195 = Reverse 1D Array(array=w362) -> (reversed array=w361:dbl[])
      n196 = Reverse 1D Array(array=w360) -> (reversed array=w359:dbl[])
      n197 = Reverse 1D Array(array=w358) -> (reversed array=w357:dbl[])
      n198 = Reverse 1D Array(array=w364) -> (reversed array=w363:dbl[])
      n199 = Reverse 1D Array(array=w356) -> (reversed array=w355:dbl[])
      n200 = Reverse 1D Array(array=w345) -> (reversed array=w344:dbl[])
      n201 = Reverse 1D Array(array=w353) -> (reversed array=w352:dbl[])
      n202 = Reverse 1D Array(array=w338) -> (reversed array=w339:dbl[])
      n203 = Reverse 1D Array(array=w337) -> (reversed array=w336:dbl[])
      n204 = Reverse 1D Array(array=w334) -> (reversed array=w333:dbl[])
      n205 = Reverse 1D Array(array=w366) -> (reversed array=w365:dbl[])
      n206 = Reverse 1D Array(array=w350) -> (reversed array=w349:dbl[])
      n207 = Reverse 1D Array(array=w343) -> (reversed array=w342:dbl[])
      n208 = Bundle(w329, w373) -> (w370:cluster{dbl[], dbl[]})  [unwired: 1 in]
      n209 = Bundle(w329, w372) -> (w371:cluster{dbl[], dbl[]})  [unwired: 1 in]
      n210 = Bundle(w329, w349) -> (→"Supply P. Thermocouple":cluster{dbl[], dbl[]})  [unwired: 1 in]
      n211 = Bundle(w329, w342) -> (→"Flow Meter Thermocouple":cluster{dbl[], dbl[]})  [unwired: 1 in]
      n212 = Bundle(w329, w339) -> (→"Inlet Thermocouple":cluster{dbl[], dbl[]})  [unwired: 1 in]
      n213 = Bundle(w329, w365) -> (→"Supply Pressure":cluster{dbl[], dbl[]})  [unwired: 1 in]
      n214 = Bundle(w329, w363) -> (→"Flow Meter Pressure":cluster{dbl[], dbl[]})  [unwired: 1 in]
      n215 = Bundle(w329, w361) -> (→"Inlet Pressure":cluster{dbl[], dbl[]})  [unwired: 1 in]
      n216 = Bundle(w329, w359) -> (→"Chamber Pressure":cluster{dbl[], dbl[]})  [unwired: 1 in]
      n217 = Bundle(w329, w357) -> (→"Vol Flow":cluster{dbl[], dbl[]})  [unwired: 1 in]
      n218 = Bundle(w329, w355) -> ()  [unwired: 1 in, 1 out]
      n219 = Bundle(w329, w383) -> ()  [unwired: 1 in, 1 out]
      n220 = Bundle(w329, w352) -> (→"AI7":cluster{dbl[], dbl[]})  [unwired: 1 in]
      n221 = Bundle(w329, w344) -> (→"Rocket Thrust":cluster{dbl[], dbl[]})  [unwired: 1 in]
      n222 = Bundle(w329, w336) -> (→"Thrust 2":cluster{dbl[], dbl[]})  [unwired: 1 in]
      n223 = Bundle(w329, w333) -> (→"Thrust 3":cluster{dbl[], dbl[]})  [unwired: 1 in]
      n224 = Build Array(w370, w371) -> (→"Process Variable vs Setpoint":cluster{dbl[], dbl[]}[])
      "Angle Sensor" <- w328
    }
  }
  n225 = local write "Ignition"(FALSE ("Ignition")) -> ()
  n226 = local write "Channel Control"(bool[] [TRUE, TRUE, TRUE, TRUE, TRUE, TRUE, TRUE, FALSE, TRUE, TRUE, FALSE, TRUE, TRUE, TRUE] ("Array")) -> ()
  n227 = local write "SP"(0.0 ("SP")) -> ()
  n228 = local write "MV"(0.0 ("MV")) -> ()
  n229 = local write "Time"(0.0 ("Time")) -> ()
  n230 = local write "PID gain schedule"(T3 [{"PID gains"={"Kc"=2.1, "Ti"=0.001, "Td"=0.0}, "max value"=0.0}, {"PID gains"={"Kc"=1.1, "Ti"=0.004, "Td"=0.0}, "max value"=180.0}, {"PID gains"={"Kc"=0.1, "Ti"=0.02, "Td"=0.0}, "max value"=200.0}]) -> ()
